vi "Create Sheet.vi"(7 "Sheet Name (Sheet1)":string="Sheet1", 8 "error in (no error)":errorcluster, 11 "Workbook Reference":refnum<k24>) -> (0 "error out":errorcluster, 2 "Sheet Reference":refnum<k24>, 3 "Workbook Reference":refnum<k24>)   [LabVIEW 2013]
uses:
  C:/PhaeronGit/LVNPOI/Resources/NPOI 2.1.1 dotnet2/NPOI.dll
  Resources/NPOI 2.1.1 dotnet2/NPOI.dll
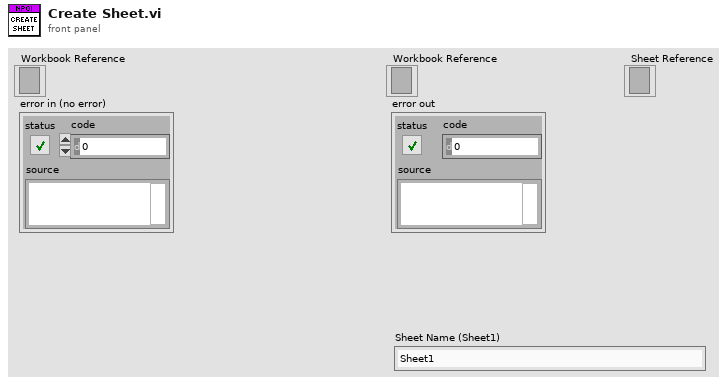
[diagram p1: front panel]
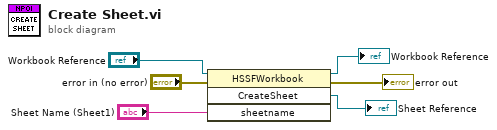
[diagram p0: block diagram]
diagram:
  n1 = invoke class="HSSFWorkbook" method="CreateSheet"(reference="Workbook Reference", error in="error in (no error)", "sheetname"="Sheet Name (Sheet1)") -> (reference out=→"Workbook Reference":refnum<k24>, error out=→"error out":errorcluster, "CreateSheet"=→"Sheet Reference":refnum<k24>)  [unwired: 1 in, 1 out]
